vi "TempLogger_w_email_v1.vi"() -> ()   [LabVIEW 2010]
uses:
  <vilib>/Utility/file.llb/Write To Spreadsheet File (DBL).vi
  <vilib>/Utility/SMTP/NI_SMTPEmail.lvlib
panel:
  in  "file path (dialog if empty)":path
  in  "Data":bool
  in  "File Path":path=path "c:/temp/email.dat"
  in  "Subject":string="Waveform Data"
  in  "Message":string="Attached is the data generated by the EMail with Data.vi"
  in  "Recipients":string[](array[string])
  in  "Mail Server":string
  in  "Return Address":string="user@test.com"
  in  "Send":bool
  in  "address":string
  in  "Port":u16
  in  "Disconnect":bool
  out "Data In":string
  in  "Mode (standard)":T1(ring)
  in  "bytes to read":i32
  out "Temperature String":string
  out "Temperature DBL":dbl
  in  "offset 1":i32
  in  "length 1":i32
  out "Temperature String 2":string
  out "Temp 2 DBL":dbl
  in  "offset 2":i32
  in  "length 2":i32
  out "initialized array":dbl[](array[numeric])
  out "Waveform Chart":dbl(graph)
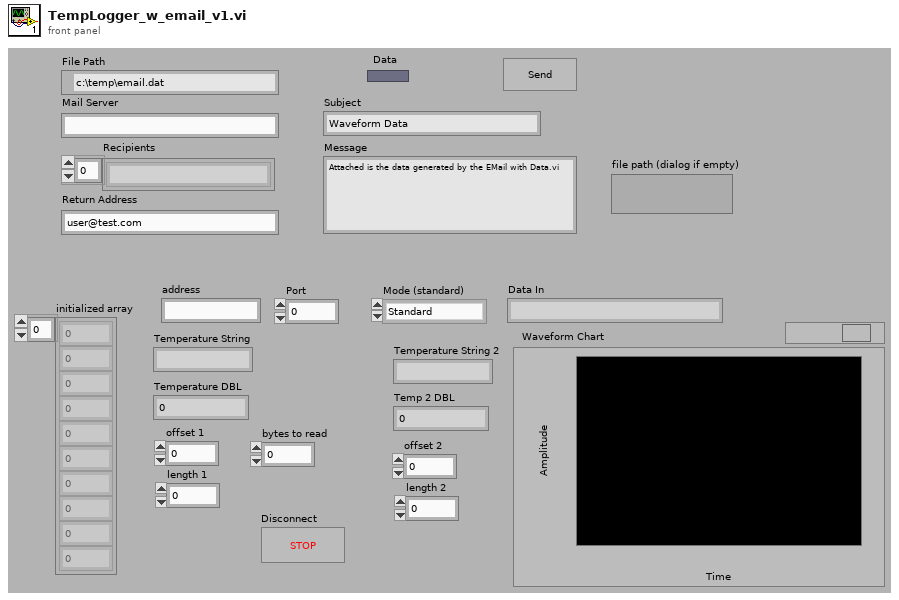
[diagram p1: front panel]
types:
  T1 = enum16{"Standard", "Buffered", "CRLF", "Immediate"}
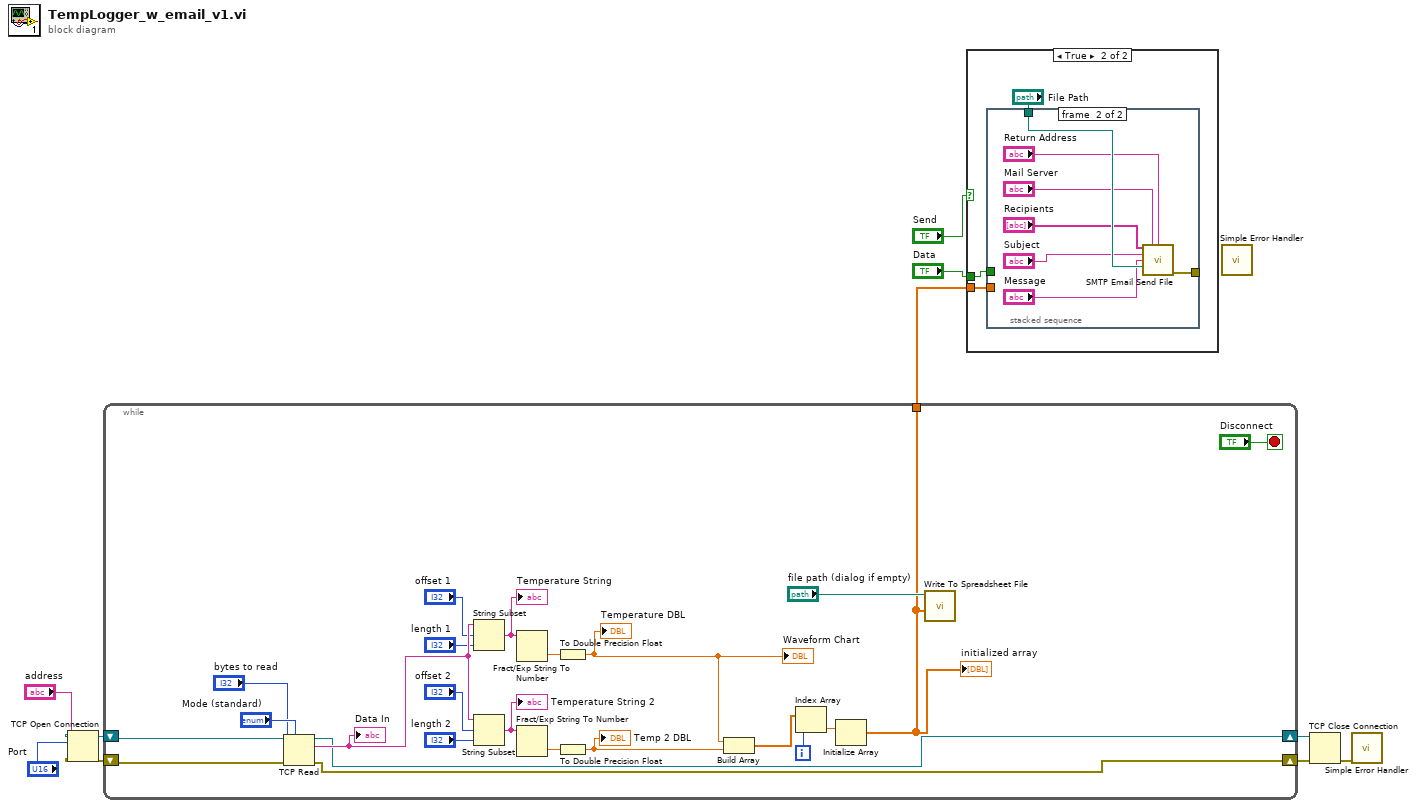
[diagram p0: block diagram]
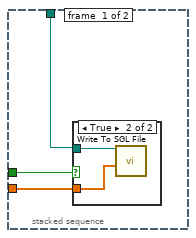
[diagram p3: hidden frame]
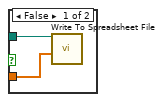
[diagram p4: hidden frame]
diagram:
  n1 = TCP Open Connection(address="address", remote port or service name="Port") -> (connection ID=w9:refnum<k5>, error out=w8:errorcluster)  [unwired: 3 in]
  n2 = while {
    shift-right: [w15] -> w6
    shift-left: w9 -> [w33]
    shift-right: [w14] -> w4
    shift-left: w8 -> [w32]
    tunnel: [w11] -> w1
    i -> [w13]
    stop <- "Disconnect" stop-if-true
    n3 = TCP Read(connection ID=w33, bytes to read="bytes to read", error in (no error)=w32, 7:"Mode (standard)") -> (connection ID out=w15:refnum<k5>, data out=w31:string, error out=w14:errorcluster)  [unwired: 1 out]
    "Data In" <- w31
    n4 = String Subset(string=w31, offset (0)="offset 1", length (rest)="length 1") -> (substring=w16:string)
    "Temperature String" <- w16
    n5 = String Subset(string=w31, offset (0)="offset 2", length (rest)="length 2") -> (substring=w18:string)
    "Temperature String 2" <- w18
    n6 = Fract/Exp String To Number(string=w16) -> (number=w23:dbl)  [unwired: 3 in, 1 out]
    n7 = Fract/Exp String To Number(string=w18) -> (number=w26:dbl)  [unwired: 3 in, 1 out]
    n8 = To Double Precision Float(number=w23) -> (double precision float=w17:dbl)
    "Temperature DBL" <- w17
    "Waveform Chart" <- w17
    n9 = To Double Precision Float(number=w26) -> (double precision float=w30:dbl)
    "Temp 2 DBL" <- w30
    n10 = Build Array "Build Array"(w17, w30) -> (w19:dbl[])
    n11 = Index Array "Index Array"(array=w19, index=w13) -> (element=w20:dbl)
    n12 = Initialize Array "Initialize Array"(w20) -> (w11:dbl[])  [unwired: 1 in]
    "initialized array" <- w11
    n13 = call-poly <vilib>:"Write To Spreadsheet File.vi"("1D data"=w11, "file path (dialog if empty)"="file path (dialog if empty)") -> ()  [unwired: 6 in, 1 out]
  }
  n14 = case shown="True" "Send" {
    tunnel: "Data" -> [_ w35]
    tunnel: w1 -> [_ w34]
    frame False {
    }
    frame True {
      n15 = stacked-sequence {
        tunnel: w34 -> [w38 _]
        tunnel: "File Path" -> [w37 w49]
        tunnel: w35 -> [w39 _]
        tunnel: [_ w50] -> _
        frame #0 {
          n16 = case shown="True" w39 {
            tunnel: w37 -> [w41 w43]
            tunnel: w38 -> [w40 w42]
            frame False {
              n17 = call-poly <vilib>:"Write To Spreadsheet File.vi"("1D data"=w40, "file path (dialog if empty)"=w41) -> ()  [unwired: 4 in, 3 out]
            }
            frame True {
              n18 = call <vilib>:"Write To SGL File.vi"("1D array"=w42, "file path (dialog if empty)"=w43) -> ()  [unwired: 2 in, 4 out]
            }
          }
        }
        frame #1 {
          n19 = call <vilib>:"SMTP Email Send File.vi"("recipients"="Recipients", "mail server"="Mail Server", "return address"="Return Address", "subject ([No Subject])"="Subject", "message"="Message", "file path"=w49) -> ("error out"=w50:errorcluster)  [unwired: 3 in, 6 out]
        }
      }
    }
  }
  n20 = call <vilib>:"Simple Error Handler.vi"() -> ()  [unwired: 2 in, 8 out]
  n21 = TCP Close Connection(connection ID=w6, error in (no error)=w4) -> (error out=w10:errorcluster)  [unwired: 2 out]
  n22 = call <vilib>:"Simple Error Handler.vi"("error in (no error)"=w10) -> ()  [unwired: 1 in, 8 out]
